vi "fill-dense-template.vi"() -> ()   [LabVIEW 2020]
uses:
  <vilib>/Analysis/7linalg.llb/Real Transpose Matrix.vi
  <vilib>/Analysis/NI_AALPro.lvlib
panel:
  in  "weight path":path
  in  "name":string
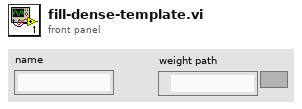
[diagram p1: front panel]
types:
  T1 = typedef "NI_Matrix.lvlib/RealMatrix.ctl" = dbl[][]
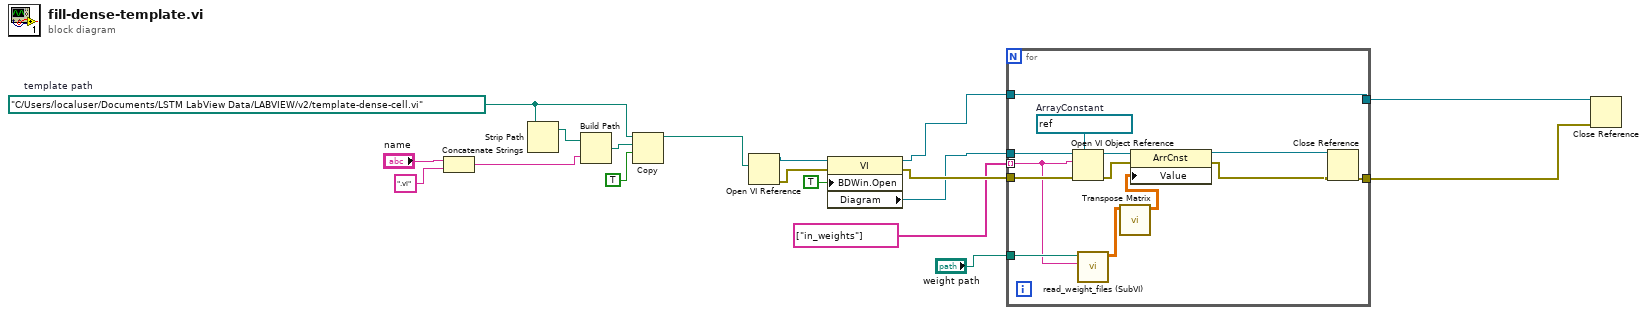
[diagram p0: block diagram]
diagram:
  w8 = path "C:/Users/localuser/Documents/LSTM LabView Data/LABVIEW/v2/template-dense-cell.vi"  # template path
  n1 = Concatenate Strings("name", ".vi") -> (w10:string)
  n2 = Strip Path(path=w8) -> (stripped path=w13:path)  [unwired: 1 out]
  n3 = Build Path(base path=w13, name or relative path=w10) -> (appended path=w9:path)
  n4 = Copy(9:TRUE, 10:w9, 11:w8) -> (3:w4:path)  [unwired: 2 in, 2 out]
  n5 = Open VI Reference(vi path=w4) -> (vi reference=w6:refnum<vi>, error out=w5:errorcluster)  [unwired: 5 in]
  n6 = property class="VI"(reference=w6, error in=w5, "BDWin.Open"=TRUE) -> (reference out=w2:refnum<vi>, error out=w15:errorcluster, "Diagram"=w3:refnum<vi>)
  n7 = for {
    tunnel: w15 -> [w31]
    tunnel: w3 -> [w30]
    tunnel: string[] ["in_weights"] -> [w25] mode=indexing
    tunnel: [w23] -> w18
    tunnel: "weight path" -> [w26]
    tunnel: [w24] -> w14
    tunnel: w2 -> [w24]
    w29 = refnum<vi> refnum  # ArrayConstant
    n8 = Open VI Object Reference(7:w29, 8:w31, 10:w25, 11:w30) -> (0:w27:errorcluster, 3:w28:refnum<vi>)
    n9 = call "read_weight_files (SubVI).vi"("weight file name"=w25, "weights path"=w26) -> ("all rows"=w20:dbl[][])  [unwired: 9 in]
    n10 = call-poly <vilib>:"Transpose Matrix.vi"("Input Matrix"=w20) -> ("Matrix Transpose"=w19:T1)  [unwired: 9 in, 1 out]
    n11 = property class="ArrCnst"(reference=w28, error in=w27, "Value"=w19) -> (reference out=w22:refnum<vi>, error out=w21:errorcluster)
    n12 = Close Reference(reference=w22, error in (no error)=w21) -> (error out=w23:errorcluster)
  }
  n13 = Close Reference(reference=w14, error in (no error)=w18) -> ()  [unwired: 1 out]
